vi "Force I32 Array To Size.vi"(5 "Default Value":dbl format="%.2f", 7 "# Elements":i32, 11 "I32 Array In":i32[](array[numeric])) -> (3 "I32 Array Out":i32[](array[numeric]))   [LabVIEW 2021]
panel:
  # "If input array has the specified number of elements, it is not changed.\nIf input array has more than the specified number of elements, the extra elements are removed from the end.\nIf input array has less than specified number of elements, it is padded using the default value."
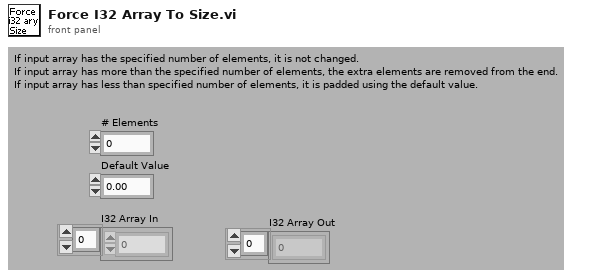
[diagram p1: front panel]
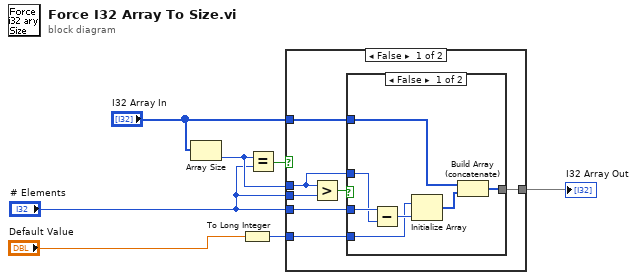
[diagram p0: block diagram]
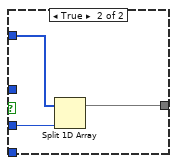
[diagram p2: hidden frame]
diagram:
  n1 = Array Size(array="I32 Array In") -> (size(s)=w7:i32)
  n2 = To Long Integer(number="Default Value") -> (32bit integer=w4:i32)
  n3 = Equal?(x=w7, y="# Elements") -> (x = y?=w6:bool)
  n4 = case shown="False" w6 {
    tunnel: w7 -> [w9 _]
    tunnel: "# Elements" -> [w14 _]
    tunnel: "# Elements" -> [w12 _]
    tunnel: "I32 Array In" -> [w11 w25]
    tunnel: [w10 w25] -> w3
    tunnel: w4 -> [w8 _]
    frame False {
      n5 = Greater?(x=w9, y=w14) -> (0:w13:bool)
      n6 = case shown="False" w13 {
        tunnel: w12 -> [w21 w24]
        tunnel: w11 -> [w16 w23]
        tunnel: [w15 w22] -> w10
        tunnel: w9 -> [w20 _]
        tunnel: w8 -> [w18 _]
        frame False {
          n7 = Subtract(x=w21, y=w20) -> (x-y=w19:i32)
          n8 = Initialize Array(w18, w19) -> (w17:i32[])
          n9 = Build Array (concatenate)(w16, w17) -> (w15:i32[])
        }
        frame True {
          n10 = Split 1D Array(array=w23, index=w24) -> (first subarray=w22:i32[])  [unwired: 1 out]
        }
      }
    }
    frame True {
    }
  }
  "I32 Array Out" <- w3
